vi "GetAnalyserPanel.vi"(8 "error in (no error)":errorcluster, 11 "Analyser in":refnum<class "Analyser.lvclass">) -> (0 "error out":errorcluster, 2 "Panel":string, 3 "Analyser out":refnum<class "Analyser.lvclass">)   [LabVIEW 2020, in "Analyser.lvlib" / "Analyser.lvclass"]
uses:
  Analyser.lvclass
  Analyser.lvclass/Analyser.ctl
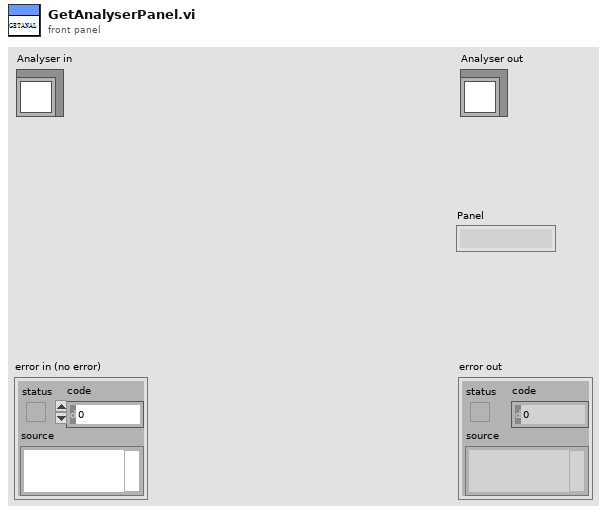
[diagram p1: front panel]
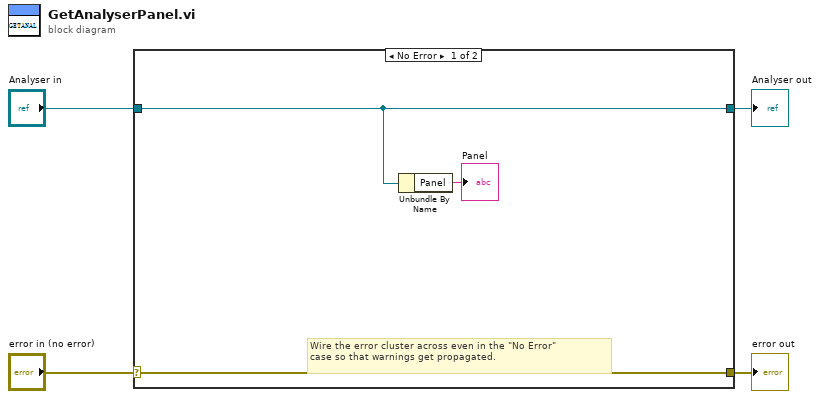
[diagram p0: block diagram]
diagram:
  n1 = case shown="No Error" "error in (no error)" {
    selector: "error in (no error)" -> [w7 w9]
    tunnel: [w7 w9] -> w3
    tunnel: [w6 w8] -> w1
    tunnel: "Analyser in" -> [w6 w8]
    frame No Error {
      # "Wire the error cluster across even in the \"No Error\"\ncase so that warnings get propagated."
      n2 = Unbundle By Name(w6) -> ("Panel"=→"Panel":string)
    }
    frame Error {
    }
  }
  "error out" <- w3
  "Analyser out" <- w1
